vi "printDocument.vi"(8 "error in (no error)":errorcluster, 10 "printer name (default)":string, 11 "MS-Word in":refnum<class "MS-Word.lvclass">) -> (0 "error out":errorcluster, 3 "MS-Word out":refnum<class "MS-Word.lvclass">)   [LabVIEW 2017, in "LabVIEW NPOI.lvlib" / "MS-Word.lvclass"]
uses:
  MS-Word.lvclass
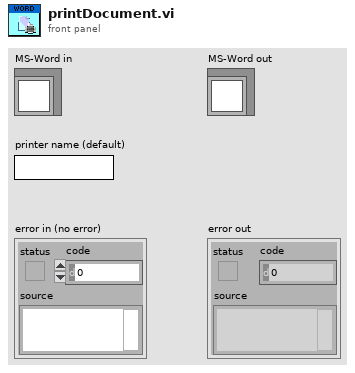
[diagram p1: front panel]
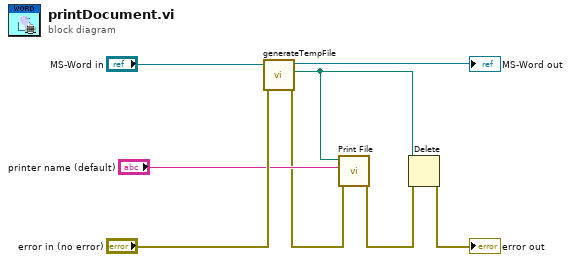
[diagram p0: block diagram]
diagram:
  n1 = call-dynamic "generateTempFile.vi"("error in (no error)"="error in (no error)", "MS-Word in"="MS-Word in") -> ("error out"=w2:errorcluster, "Temporary File Path"=w8:path, "MS-Word out"=→"MS-Word out":refnum<class "MS-Word.lvclass">)  [unwired: 7 in]
  n2 = call "Print File.vi"("error in (no error)"=w2, "Printer Name (default)"="printer name (default)", "File Path"=w8) -> ("error out"=w3:errorcluster)  [unwired: 7 in, 1 out]
  n3 = Delete(path (use dialog)=w8, error in=w3) -> (error out=→"error out":errorcluster)  [unwired: 3 in, 2 out]
